vi "test Get RX Mappables2.vi"(11 "Test Case In":refnum<class "Test PDO Mapping.lvclass">) -> (0 "error out":errorcluster, 3 "Test Case Out":refnum<class "Test PDO Mapping.lvclass">)   [LabVIEW 2020, in "Test PDO Mapping.lvclass"]
uses:
  Test PDO Mapping.lvclass
  C:/Program Files/National Instruments/LabVIEW 2026/vi.lib/Astemes/LUnit/Test Case.lvclass
  EDS-File-Viewer/source/Electronic Datasheet/Electronic Datasheet.lvclass/Electronic Datasheet.ctl
  <vilib>/Astemes/LUnit/Test Case.lvclass/Test Case.ctl
  4993e8ee-a06a-463a-9684-69129f64d5ce.vi
  EDS-File-Viewer/source/Electronic Datasheet/Electronic Datasheet.lvclass
  source/CANopen.lvlib
  source/Typedefs/Data Type.ctl
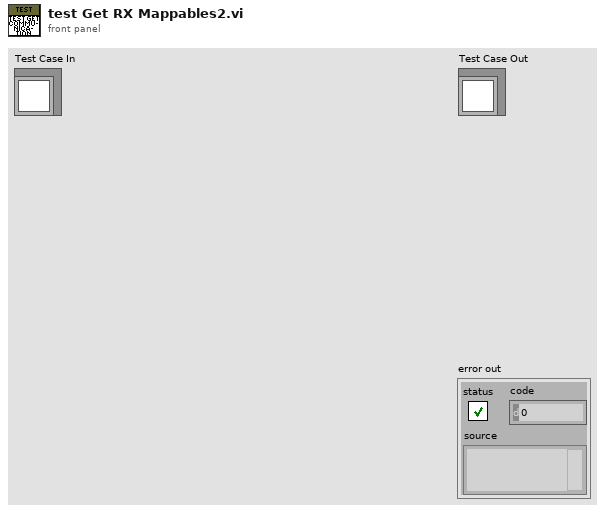
[diagram p1: front panel]
types:
  T1 = typedef "CANopen.lvlib/Data Type.ctl" = u16
  T2 = cluster{"Index":u16, "Sub Index":u8, "Name":string, "Data Type":T1}[]
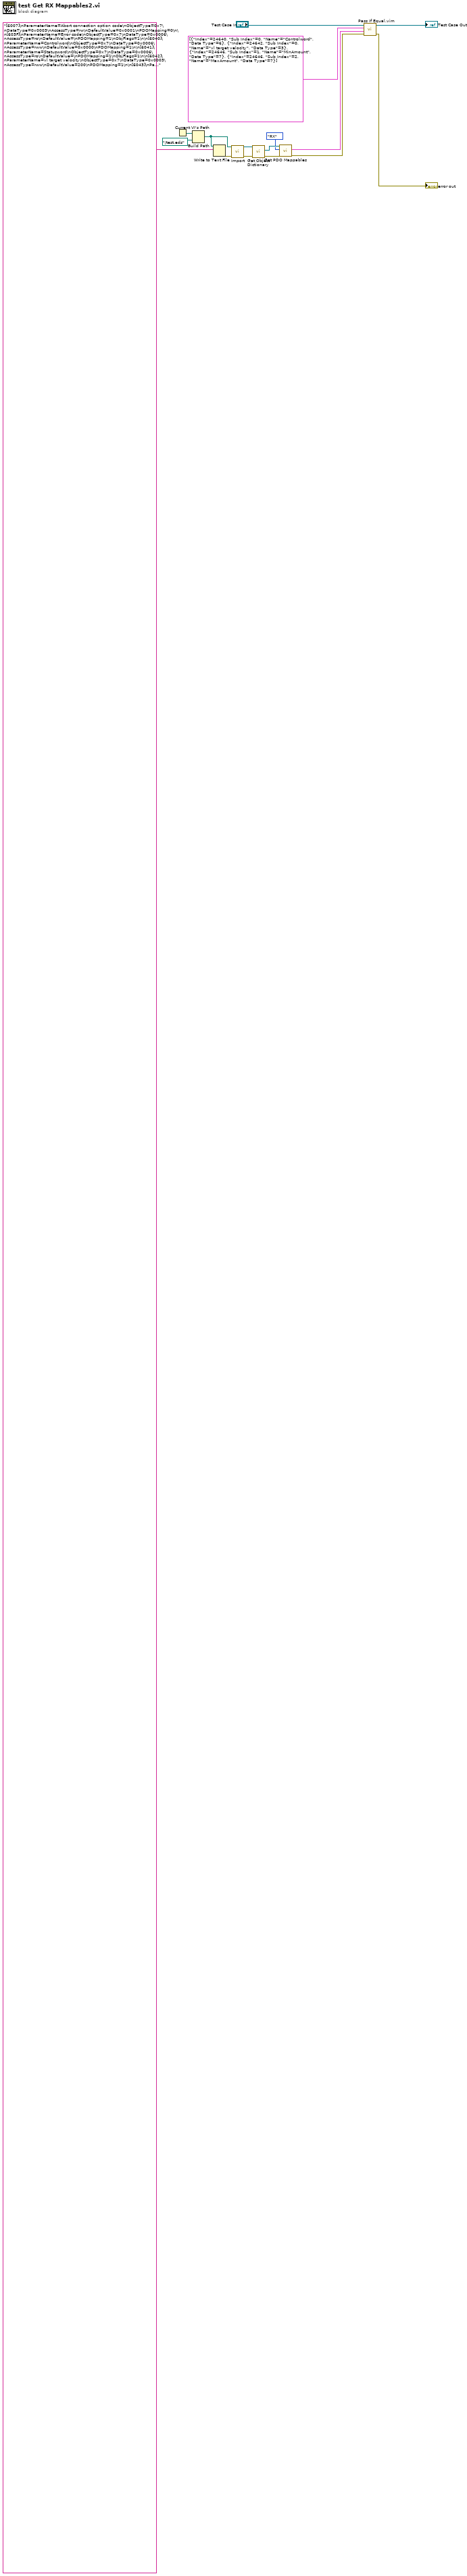
[diagram p0: block diagram]
diagram:
  n1 = Current VI's Path() -> (path=w13:path)
  n2 = Build Path(base path=w13, name or relative path=path "../test.eds") -> (appended path=w10:path)
  n3 = Write to Text File(file (use dialog)=w10, text="[6007]\nParameterName=Abort connection option code\nObjectType=0x7\nDataType=0x0003\nAccessType=rw\nDefaultValue=0x0001\nPDOMapping=0\n\n[603F]\nParameterName=Error code\nObjectType=0x7\nDataType=0x0006\nAccessType=ro\nDefaultValue=\nPDOMapping=1\nObjFlags=1\n\n[6040]\nParameterName=Controlword\nObjectType=0x7\nDataType=0x0006\nAccessType=rww\nDefaultValue=0x0000\nPDOMapping=1\n\n[6041]\nParameterName=Statusword\nObjectType=0x7\nDataType=0x0006\nAccessType=ro\nDefaultValue=\nPDOMapping=1\nObjFlags=1\n\n[6042]\nParameterName=vl target velocity\nObjectType=0x7\nDataType=0x0003\nAccessType=rww\nDefaultValue=200\nPDOMapping=1\n\n[6043]\nParameterName=vl velocity demand\nObjectType=0x7\nDataType=0x0003\nAccessType=ro\nDefaultValue=0x0000\nPDOMapping=1\nObjFlags=1\n\n[6044]\nParameterName=vl velocity actual value\nObjectType=0x7\nDataType=0x0003\nAccessType=ro\nDefaultValue=0x0000\nPDOMapping=1\nObjFlags=1\n\n[6046]\nParameterName=vl velocity min max amount\nObjectType=0x8\nSubNumber=0x03\n\n[6046sub0]\nParameterName=Number of entries\nObjectType=0x7\nDataType=0x0005\nAccessType=const\nDefaultValue=2\nPDOMapping=0\n\n[6046sub1]\nParameterName=MinAmount\nObjectType=0x7\nDataType=0x0007\nAccessType=rww\nDefaultValue=0\nPDOMapping=1\n\n[6046sub2]\nParameterName=MaxAmount\nObjectType=0x7\nDataType=0x0007\nAccessType=rww\nDefaultValue=30000\nPDOMapping=1") -> (error out=w9:errorcluster)  [unwired: 2 in, 2 out]
  n4 = call "Import.vi"("error in"=w9, "EDS File Path"=w10) -> ("error out"=w8:errorcluster, "Electronic Datasheet"=w6:refnum<class "Electronic Datasheet.lvclass">)  [unwired: 8 in]
  n5 = call "Get Object Dictionary.vi"("error in"=w8, "Electronic Datasheet in"=w6) -> ("error out"=w7:errorcluster, "Obj Dict"=w5:refnum<class "Object Dictionary.lvclass">)  [unwired: 7 in, 1 out]
  n6 = call "Get PDO Mappables.vi"("error in"=w7, "Type"=enum16{"RX", "TX"}."RX", "Object Dictionary in"=w5) -> ("error out"=w4:errorcluster, "PDO Mappables"=w2:T2)  [unwired: 6 in, 1 out]
  n7 = call "Pass If Equal.vim"("error in (no error)"=w4, "Actual"=w2, "Expected"=T2 [{"Index"=24640, "Sub Index"=0, "Name"="Controlword", "Data Type"=6}, {"Index"=24642, "Sub Index"=0, "Name"="vl target velocity", "Data Type"=3}, {"Index"=24646, "Sub Index"=1, "Name"="MinAmount", "Data Type"=7}, {"Index"=24646, "Sub Index"=2, "Name"="MaxAmount", "Data Type"=7}] ("PDO Mappables"), "LUnit Test Case In"="Test Case In") -> ("error out"=→"error out":errorcluster, "LUnit Test Case Out"=→"Test Case Out":refnum<class "Test PDO Mapping.lvclass">)  [unwired: 6 in]
